vi "CSM - Replace Mark with String Array.vi"(0 "Single-line Text":string="All Data Saved@TDMS >> API: Terminate@<1> -><register>", 5 "Replace String":string[](array[string]), 9 "Substitution Mark":enum16{"<1>", "<2>", "<3>", "<4>"}(ring)) -> (4 "States":string)   [LabVIEW 2017, in "Communicable State Machine.lvlib"]
doc: "Replaces tags in a single state string with strings from an array and merges them into a string describing a group of states.\n\n<b>Example</b>: For `Draw >> <1> -@ Painter`, <b>Tag</b> should be set to `<1>`\n\nInput array `[Line, Circle, Rectangle]`. The result will be:\n\n Draw >> Line -@ Painter\n Draw >> Circle -@ Painter\n Draw >> Rectangle -@ Painter\n\n-- <b>Controls</b> --\n- <b>single-line text</b>: Single-line state string containing tags like `<1>`, `<2>`, `<3>`, etc.\n- <b>Substitution Mark</b>: The tag to replace, such as `<1>`, `<2>`, `<3>`, etc.\n- <b>replace string</b>: The array of strings to replace the tag with.\n\n-- <b>Indicators</b> --\n- <b>States</b>: The merged state string."
uses:
  Communicable State Machine.lvlib
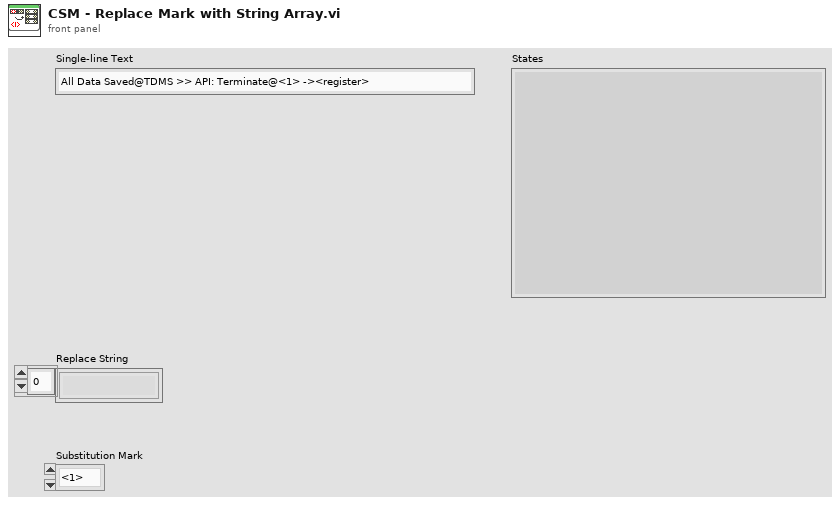
[diagram p1: front panel]
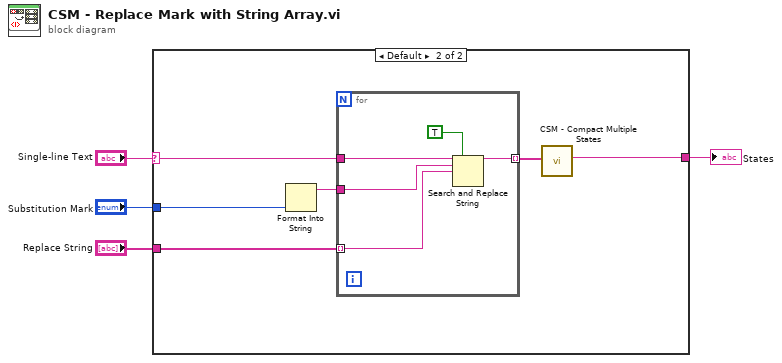
[diagram p0: block diagram]
diagram:
  n1 = case shown="Default" "Single-line Text" {
    selector: "Single-line Text" -> [_ w7]
    tunnel: [_ w10] -> w4
    tunnel: "Replace String" -> [_ w8]
    tunnel: "Substitution Mark" -> [_ w6]
    frame "" {
    }
    frame Default {
      n2 = Format Into String(w6) -> (resulting string=w5:string)  [unwired: 3 in, 1 out]
      n3 = for {
        tunnel: w7 -> [w15]
        tunnel: w8 -> [w13] mode=indexing
        tunnel: [w12] -> w9 mode=indexing
        tunnel: w5 -> [w11]
        n4 = Search and Replace String(replace all?=TRUE ("replace all? (F)"), input string=w15, search string=w11, replace string=w13) -> (result string=w12:string)  [unwired: 4 in, 3 out]
      }
      n5 = call "CSM - Compact Multiple States.vi"("Multiple States"=w9) -> ("States"=w10:string)  [unwired: 9 in]
    }
  }
  "States" <- w4
